vi "ReadFromDigi.vi"(7 "Timeout (ms)":i32=-1, 8 "error in":errorcluster, 9 "Number of Elements":u32, 10 "Mode":enum16{"Wait For Data", "Timeout"}(ring)=enum."Timeout", 11 "FPGA VI Reference":T1) -> (0 "error out":errorcluster, 1 "Error/Timeout?":bool, 2 "Output Waveform":u16[](array[numeric]), 3 "FPGA VI Reference Out":T1)   [LabVIEW 2020]
uses:
  DigiFPGARef.ctl
  <vilib>/Utility/error.llb/Error Cluster From Error Code.vi
  <vilib>/rvi/errors/niLvFpgaAdjustHostInterfaceError.vi
  <vilib>/rvi/interface/nirviMethod/nirviMethod.xnode
  <vilib>/FPGAPlugInAG/Dynamic/niLvFpga_ReadFifo_Dynamic.vi
  <vilib>/rvi/errors/niLvFpgaMergeErrorWithErrorCode.vi
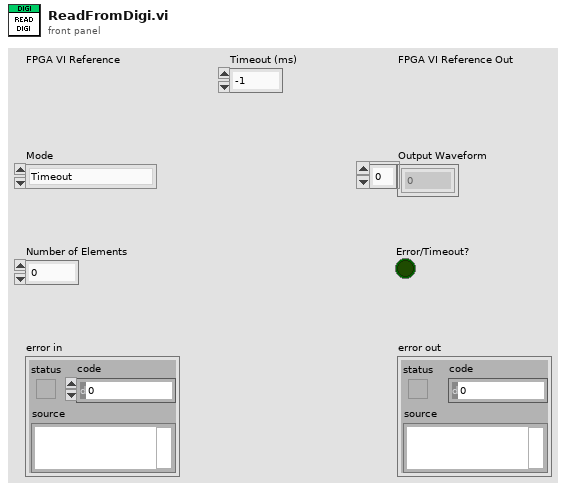
[diagram p1: front panel]
types:
  T1 = typedef "DigiFPGARef.ctl" = refnum<k20>
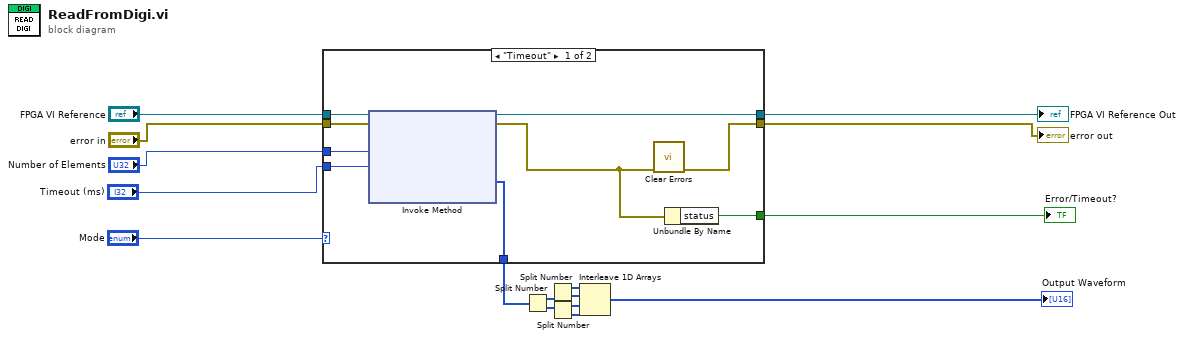
[diagram p0: block diagram]
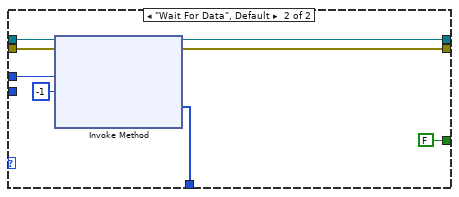
[diagram p2: hidden frame]
diagram:
  n1 = case shown="\"Timeout\"" "Mode" {
    tunnel: [w25 w33] -> w16
    tunnel: "Timeout (ms)" -> [w24 _]
    tunnel: "FPGA VI Reference" -> [w23 w32]
    tunnel: [w22 w31] -> w7
    tunnel: [w19 w30] -> w6
    tunnel: "error in" -> [w21 w29]
    tunnel: "Number of Elements" -> [w20 w27]
    tunnel: [w17 FALSE ("status")] -> w2
    frame "Timeout" {
      n2 = xnode "Invoke Method"("FPGA VI Reference In"=w23, "error in"=w21, "Number of Elements"=w20, "Timeout (ms)"=w24) -> ("FPGA VI Reference Out"=w22:T1, "error out"=w18:errorcluster, "Data"=w25:u64[])  [unwired: 1 out]
      n3 = call <vilib>:"Clear Errors.vi"("error in (no error)"=w18) -> ("error out"=w19:errorcluster)  [unwired: 5 in, 1 out]
      n4 = Unbundle By Name(w18) -> ("status"=w17:bool)
    }
    frame "Wait For Data", Default {
      n5 = xnode "Invoke Method"("FPGA VI Reference In"=w32, "error in"=w29, "Number of Elements"=w27, "Timeout (ms)"=-1) -> ("FPGA VI Reference Out"=w31:T1, "error out"=w30:errorcluster, "Data"=w33:u64[])  [unwired: 1 out]
    }
  }
  "error out" <- w6
  "FPGA VI Reference Out" <- w7
  "Error/Timeout?" <- w2
  n6 = Split Number(x=w16) -> (hi(x)=w14:u32[], lo(x)=w13:u32[])
  n7 = Split Number(x=w14) -> (hi(x)=w12:u16[], lo(x)=w9:u16[])
  n8 = Split Number(x=w13) -> (hi(x)=w10:u16[], lo(x)=w11:u16[])
  n9 = Interleave 1D Arrays(w12, w9, w10, w11) -> (→"Output Waveform":u16[])
